vi "reduce_size_waveform.vi"(1 "Waveform Data IN":waveform(dbl)[](graph)) -> (0 "Waveform Data OUT":waveform(dbl)[](graph))   [LabVIEW 2018]
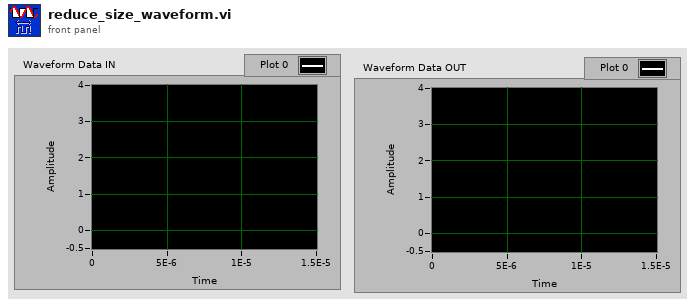
[diagram p1: front panel]
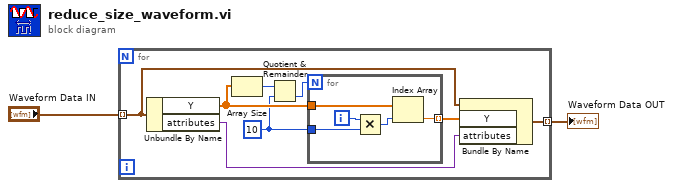
[diagram p0: block diagram]
diagram:
  n1 = for {
    tunnel: "Waveform Data IN" -> [w10] mode=indexing
    tunnel: [w8] -> w1 mode=indexing
    w4 = 10 ("y")
    n2 = Unbundle By Name(w10) -> ("Y"=w5:dbl[], "attributes"=w9:variant)
    n3 = Array Size(array=w5) -> (size(s)=w7:i32)
    n4 = Quotient & Remainder(x=w7, y=w4) -> (floor(x/y)=w6:i32)  [unwired: 1 out]
    n5 = for {
      N: w6 -> [_]
      tunnel: w5 -> [w15]
      tunnel: w4 -> [w13]
      tunnel: [w11] -> w3 mode=indexing
      i -> [w14]
      n6 = Multiply(x=w14, y=w13) -> (x*y=w12:i32)
      n7 = Index Array(array=w15, index=w12) -> (element=w11:dbl)
    }
    n8 = Bundle By Name(cluster=w10, "Y"=w3, "attributes"=w9) -> (w8:waveform(dbl))
  }
  "Waveform Data OUT" <- w1
